vi "Deplacement avant-recul.vi"() -> ()   [LabVIEW 2019]
uses:
  <vilib>/addons/control/pid/NI_PID_pid.lvlib
  <vilib>/addons/control/pid/pid.llb/PID (DBL).vi
  Global.vi
  <vilib>/Rock Robotics/WPI/ThirdParty/Phoenix-LabVIEW/Motor Controller/Get/CTRE_Phoenix_MotorController_GetQuadratureData.vi
panel:
  in  "Deplacement (m)":dbl
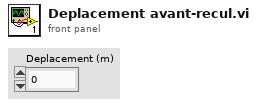
[diagram p1: front panel]
types:
  T1 = cluster{"proportional gain (Kc)":dbl, "integral time (Ti, min)":dbl, "derivative time (Td, min)":dbl}
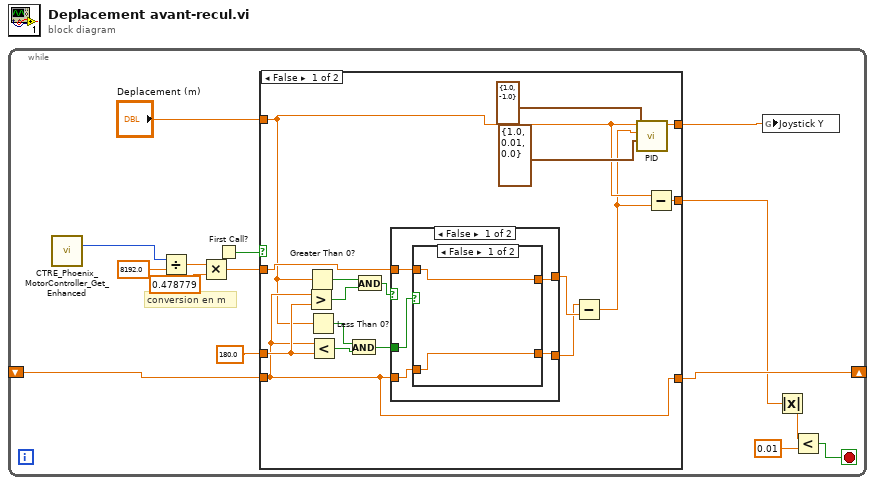
[diagram p0: block diagram]
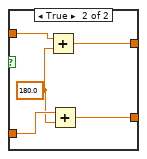
[diagram p2: hidden frame]
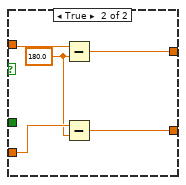
[diagram p3: hidden frame]
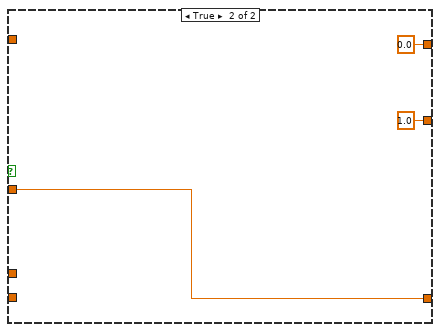
[diagram p4: hidden frame]
diagram:
  n1 = while {
    shift-right: [w14] -> _
    shift-left: _ -> [w13]
    stop <- w9 stop-if-true
    # "conversion en m"
    n2 = call-poly <vilib>:"CTRE_Phoenix_MotorController_Get_Enhanced.vi"() -> ("Quadrature Position"=w1:i32)  [unwired: 12 in, 3 out]
    n3 = Divide(x=w1, y=8192.0) -> (x/y=w5:dbl)
    n4 = Multiply(x=w5, y=0.478779) -> (x*y=w3:dbl)
    n5 = First Call?() -> (First Call?: T/F=w15:bool)
    n6 = case shown="False" w15 {
      tunnel: w3 -> [w23 w52]
      tunnel: [w20 w52] -> w14
      tunnel: w13 -> [w20 _]
      tunnel: "Deplacement (m)" -> [w18 _]
      tunnel: 180.0 ("x") -> [w26 _]
      tunnel: [w19 0.0 ("output")] -> w10
      tunnel: [w16 1.0] -> w8
      frame False {
        n7 = Greater?(x=w20, y=w26) -> (0:w27:bool)
        n8 = Greater Than 0?(x=w18) -> (x > 0?=w28:bool)
        n9 = Less Than 0?(x=w18) -> (x < 0?=w29:bool)
        n10 = Less?(x=w20, y=w26) -> (x < y?=w30:bool)
        n11 = And(x=w29, y=w30) -> (x .and. y?=w24:bool)
        n12 = And(x=w28, y=w27) -> (x .and. y?=w25:bool)
        n13 = case shown="False" w25 {
          tunnel: w24 -> [w37 _]
          tunnel: w23 -> [w35 w48]
          tunnel: w20 -> [w36 w49]
          tunnel: [w33 w46] -> w21
          tunnel: [w34 w45] -> w22
          frame False {
            n14 = case shown="False" w37 {
              tunnel: w36 -> [w39 w44]
              tunnel: w35 -> [w38 w43]
              tunnel: [w38 w41] -> w34
              tunnel: [w39 w40] -> w33
              frame False {
              }
              frame True {
                w42 = 180.0 ("y")
                n15 = Add(x=w43, y=w42) -> (x+y=w41:dbl)
                n16 = Add(x=w44, y=w42) -> (x+y=w40:dbl)
              }
            }
          }
          frame True {
            w47 = 180.0 ("y")
            n17 = Subtract(x=w48, y=w47) -> (x-y=w45:dbl)
            n18 = Subtract(x=w49, y=w47) -> (x-y=w46:dbl)
          }
        }
        n19 = Subtract(x=w21, y=w22) -> (x-y=w17:dbl)
        n20 = call-poly <vilib>:"PID.vi"("output range"=cluster{"output high":dbl, "output low":dbl} {"output high"=1.0, "output low"=-1.0}, "PID gains"=T1 {"proportional gain (Kc)"=1.0, "integral time (Ti, min)"=0.01, "derivative time (Td, min)"=0.0}, "process variable"=w17, "setpoint"=w18) -> ("output"=w19:dbl)  [unwired: 6 in, 1 out]
        n21 = Subtract(x=w18, y=w17) -> (x-y=w16:dbl)
      }
      frame True {
      }
    }
    n22 = global write "Global.vi" "Joystick Y"(w10) -> ()
    n23 = Absolute Value(x=w8) -> (abs(x)=w6:dbl)
    n24 = Less?(x=w6, y=0.01) -> (x < y?=w9:bool)
  }
